vi "Check for CAN Error Gen.vi"(9 "ID ERROR MESSAGE":u32=255 format="%x", 10 "payload":u8[](array[numeric]), 11 "identifier":u32) -> (2 "Error Number":u8, 3 "Error":bool)   [LabVIEW 2025]
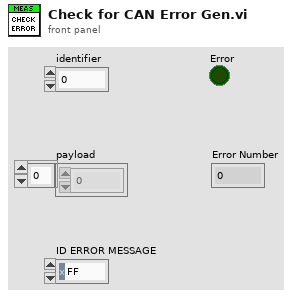
[diagram p1: front panel]
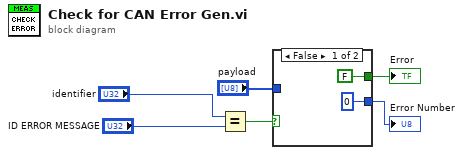
[diagram p0: block diagram]
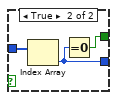
[diagram p2: hidden frame]
diagram:
  n1 = Equal?(x="identifier", y="ID ERROR MESSAGE") -> (x = y?=w4:bool)
  n2 = case shown="False" w4 {
    tunnel: "payload" -> [_ w11]
    tunnel: [FALSE w10] -> w2
    tunnel: [u8 0 ("Numeric") w9] -> w1
    frame False {
    }
    frame True {
      n3 = Index Array(array=w11) -> (element=w9:u8)  [unwired: 1 in]
      n4 = Equal To 0?(x=w9) -> (x = 0?=w10:bool)
    }
  }
  "Error" <- w2
  "Error Number" <- w1
